vi "Create Name Refs.vi"(6 "Name":string, 8 "error in":errorcluster, 9 "Name Library File Path":path, 10 "Active Project":refnum<vi>) -> (0 "error out":errorcluster, 2 "Name Refs":T1)   [LabVIEW 2025, in "_Rescript.lvlib" / "Msg.lvlib" / "Msg.lvclass"]
uses:
  _Rescript/_Rescript.lvclass/_Rescript.ctl
  Msg.lvclass
  Msg.lvclass/Msg.ctl
  Name jettl Msg.ctl
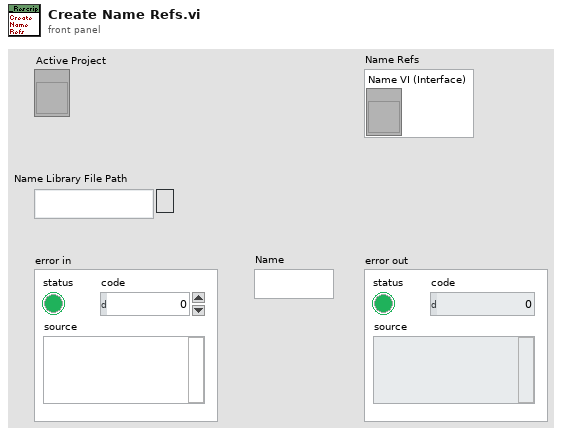
[diagram p1: front panel]
types:
  T1 = typedef "_Rescript.lvlib/Msg.lvlib/Msg.lvclass/Name jettl Msg.ctl" = cluster{"Name VI (Interface)":refnum<vi>}
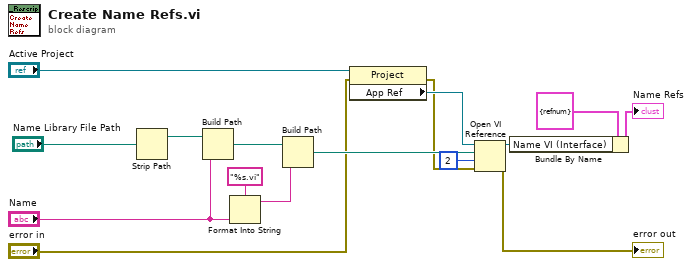
[diagram p0: block diagram]
diagram:
  n1 = Strip Path(path="Name Library File Path") -> (stripped path=w9:path)  [unwired: 1 out]
  n2 = Build Path(base path=w9, name or relative path="Name") -> (appended path=w16:path)
  n3 = Format Into String(format string="%s.vi", "Name") -> (resulting string=w15:string)  [unwired: 2 in, 1 out]
  n4 = Build Path(base path=w16, name or relative path=w15) -> (appended path=w13:path)
  n5 = property class="Project"(reference="Active Project", error in="error in") -> (error out=w2:errorcluster, "App Ref"=w3:refnum<vi>)  [unwired: 1 out]
  n6 = Open VI Reference(application reference (local)=w3, vi path=w13, options=2, error in (no error)=w2) -> (vi reference=w6:refnum<vi>, error out=→"error out":errorcluster)  [unwired: 2 in]
  n7 = Bundle By Name(cluster=T1 {"Name VI (Interface)"=refnum} ("Name Refs"), "Name VI (Interface)"=w6) -> (→"Name Refs":T1)
